vi "Main - Process Cluster.vi"() -> (0 "Cluster":T1)   [LabVIEW 2011]
doc: "This VI holds the cluster information for the Queue Driven Message Handler (QDMH). Once the QDMH has been created, this should also be saved as a new VI.\n\nAAL 9/09"
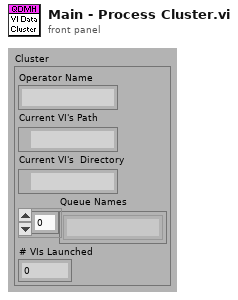
[diagram p1: front panel]
types:
  T1 = cluster{"Operator Name":string, "Current VI's Path":path, "Current VI's  Directory":path, "Queue Names":string[], "# VIs Launched":i32}
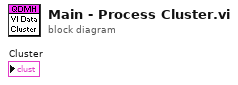
[diagram p0: block diagram]
diagram:
